vi "Configure Connection Dialog.vi"(8 "error in (no error)":errorcluster, 10 "Current Connection":T8, 11 "Channel Editor State":T1={"Modules and Connections"=[{" Module Path"="", "Short Module Path"="", "Product Name"="", "Possible Connections"=[], "Missing"=FALSE}, {" Module Path"="", "Short Module Path"="", "Product Name"="", "Possible Connections"=[], "Missing"=FALSE}], "Alias Mappings UI"=[], "Mappings by Module UI"=[]}) -> (0 "error out":errorcluster, 1 "Connection (R,S,D)":T7, 2 "Canceled?":bool)   [LabVIEW 2020, in "Routing and Faulting System Explorer.lvlib"]
uses:
  Routing and Faulting System Explorer.lvlib
  Connection Row.ctl
  Shared/Connection.ctl
  Channel Editor State.ctl
  Possible Connections.ctl
  Shared/Routing and Faulting Hardware API/Types/Possible Connections for Endpoint.ctl
  Shared/Alias Mapping.ctl
  Shared/Alias Endpoint.ctl
  Alias Map by Module.ctl
  <vilib>/event_ctls.llb/lveventtype.ctl
  Shared/Constants.vi
  Shared/Routing and Faulting Shared.lvlib
  Shared/Routing and Faulting Hardware API/Routing and Faulting Hardware API.lvlib
panel:
  out "Product Name List":string[](array[string])
  out "Module Index":i32
  out "Initial Module":string
  out "Initial Destination":string
  out "Initial Source":string
  in  "Module":string(combo)
  in  "Cancel Button":bool
  in  "OK Button":bool
  in  "Destination":string(combo)
  in  "Source":string(combo)
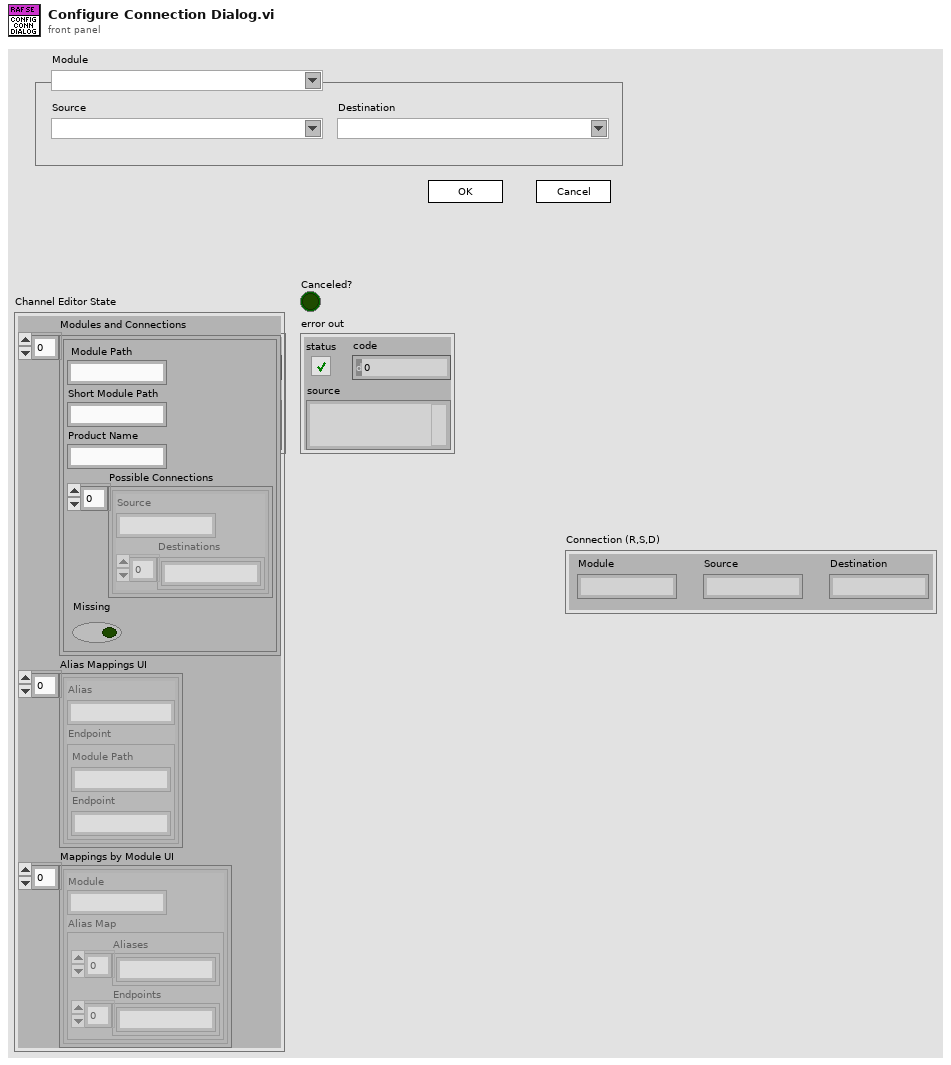
[diagram p1: front panel]
types:
  T1 = typedef "Routing and Faulting System Explorer.lvlib/Channel Editor State.ctl" = cluster{"Modules and Connections":T2[], "Alias Mappings UI":T4[], "Mappings by Module UI":T6[]}
  T2 = typedef "Routing and Faulting System Explorer.lvlib/Possible Connections.ctl" = cluster{" Module Path":string, "Short Module Path":string, "Product Name":string, "Possible Connections":T3[], "Missing":bool}
  T3 = typedef "Routing and Faulting Hardware API.lvlib/Possible Connections for Endpoint.ctl" = cluster{"Source":string, "Destinations":string[]}
  T4 = typedef "Routing and Faulting Shared.lvlib/Alias Mapping.ctl" = cluster{"Alias":string, "Endpoint":T5}
  T5 = typedef "Routing and Faulting Shared.lvlib/Alias Endpoint.ctl" = cluster{"Module Path":string, "Endpoint":string}
  T6 = typedef "Routing and Faulting System Explorer.lvlib/Alias Map by Module.ctl" = cluster{"Module":string, "Alias Map":cluster{"Aliases":string[], "Endpoints":string[]}}
  T7 = typedef "Routing and Faulting Shared.lvlib/Connection.ctl" = cluster{"Module":string, "Source":string, "Destination":string}
  T8 = typedef "Routing and Faulting System Explorer.lvlib/Connection Row.ctl" = cluster{"Source":string, "Destination":string, "Edit":bool, "Remove":bool}
  T9 = typedef "lveventtype.ctl" = enum32{"Null", "Timeout", "Annotation Menu Selection", "Annotation Menu Selection?", "App Instance Close", "App Instance Close?", "Autoscale Range Change", "Bookmark Info Change", "Cell Edit", "Cell Edit?", "Cursor Grab", "Cursor Grab?", "Cursor Menu Selection", "Cursor Menu Selection?", "Cursor Move", "Cursor Release", "Data Change", "Direction Change", "Display State Change", "Drag Ended", "Drag Enter", "Drag Leave", "Drag Over", "Drag Source Update", "Drag Starting", "Drag Starting?", "Drop", "Exec State Change", "Key Down", "Key Down?", "Key Repeat", "Key Repeat?", "Key Up", "Listbox Double Click", "Menu Activation?", "Menu Selection (App)", "Menu Selection? (App)", "Menu Selection (User)", "Mouse Down", "Mouse Down?", "Mouse Enter", "Mouse Leave", "Mouse Move", "Mouse Up", "Mouse Wheel", "NI Security User Change (App)", "Pane Size", "Panel Close", "Panel Close?", "Panel Resize", "Plot Attribute Change", "Scale Range Change", "Shortcut Menu Activation?", "Shortcut Menu Selection (App)", "Shortcut Menu Selection? (App)", "Shortcut Menu Selection (User)", "Tree Double Click", "Tree Drag", "Tree Drag?", "Tree Drop", "Tree Drop?", "Tree Item Close", "Tree Item Close?", "Tree Item Open", "Tree Item Open?", "User Event", "Value Change"}
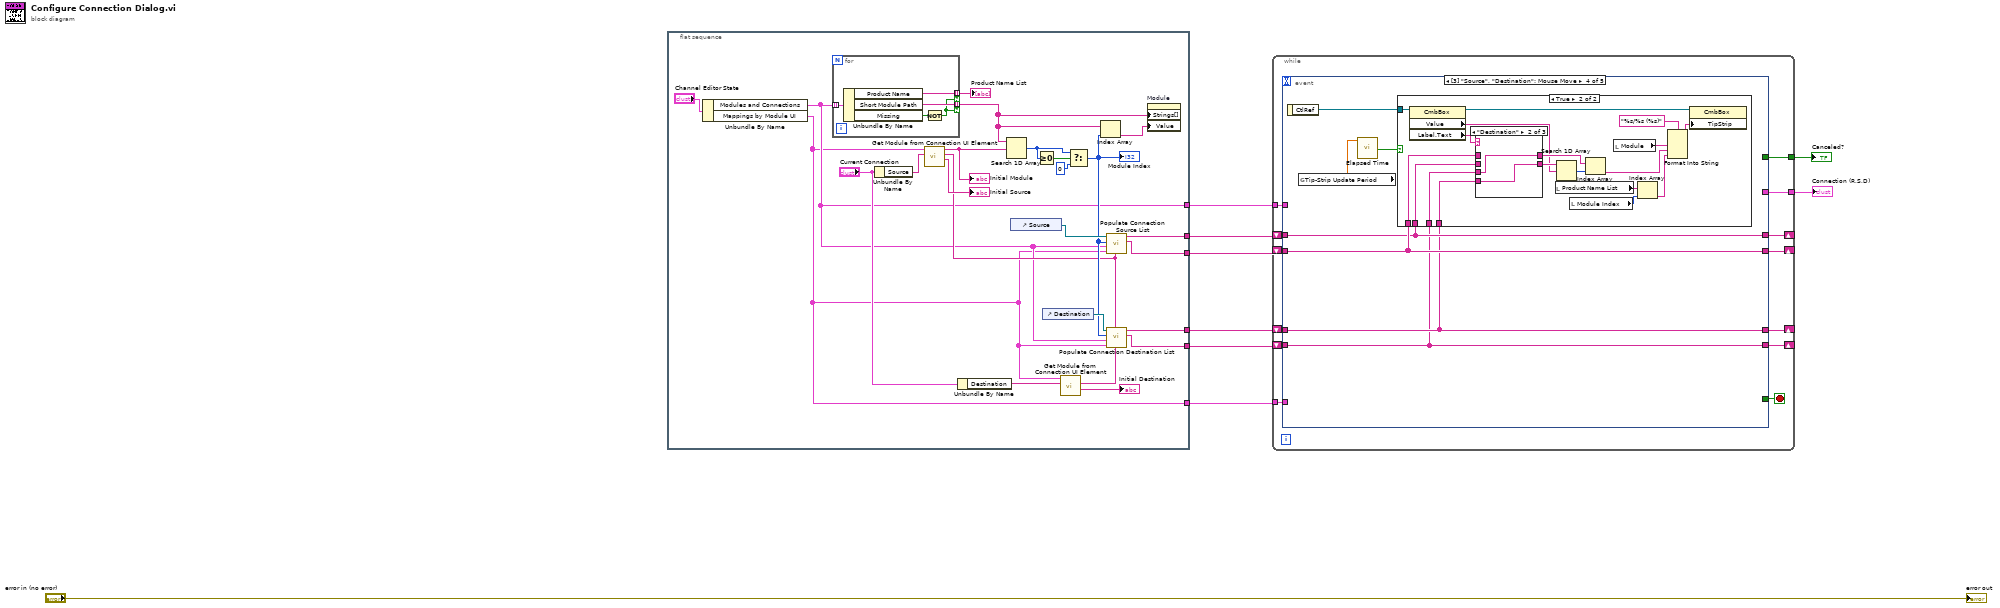
[diagram p0: block diagram]
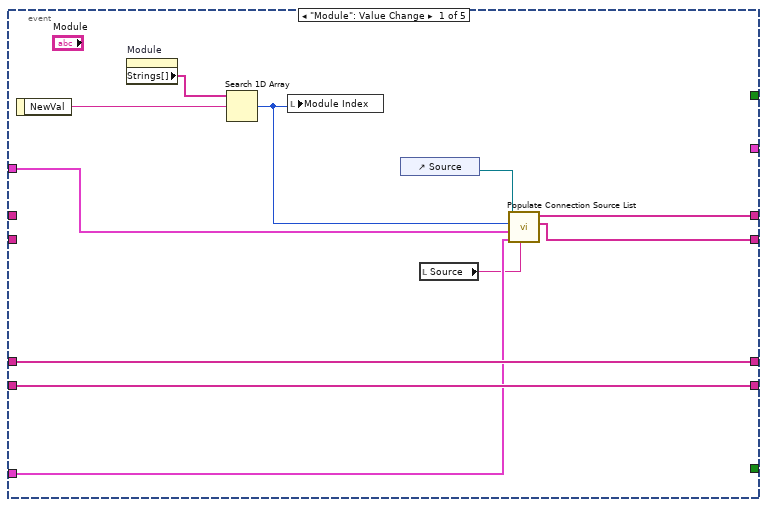
[diagram p2: hidden frame]
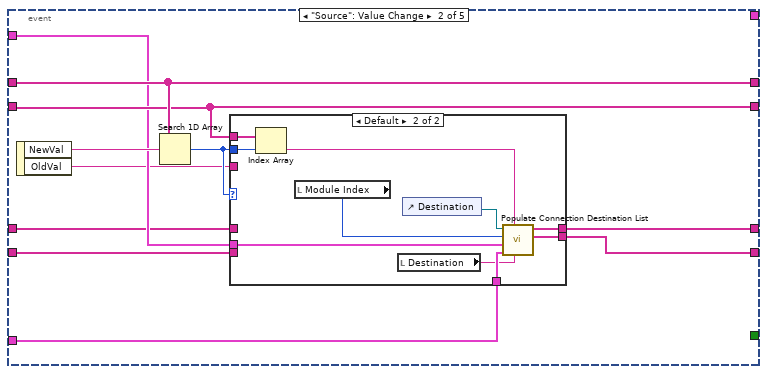
[diagram p3: hidden frame]
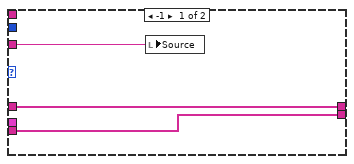
[diagram p4: hidden frame]
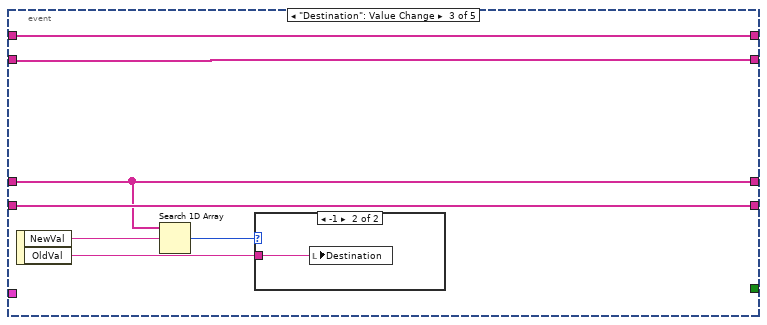
[diagram p5: hidden frame]
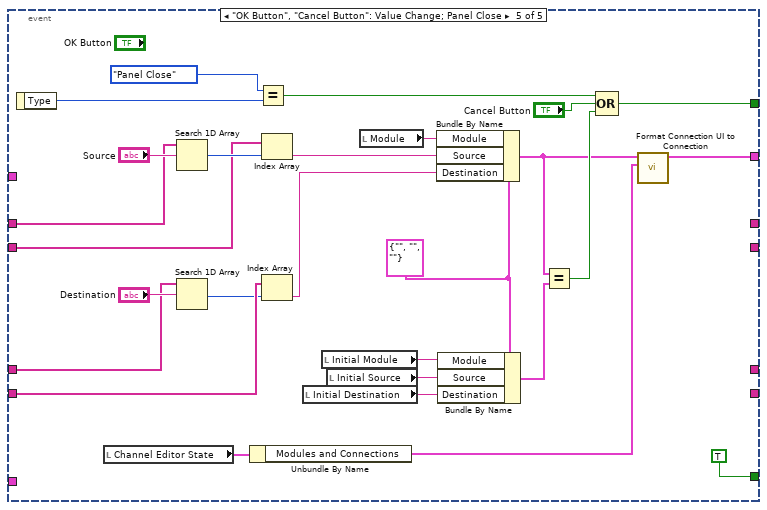
[diagram p10: hidden frame]
diagram:
  n1 = flat-sequence {
    tunnel: [w29] -> w7
    tunnel: [w11] -> w2
    tunnel: [w26] -> w6
    tunnel: [w25] -> w5
    tunnel: [w12] -> w4
    tunnel: [w28] -> w3
    frame #0 {
      n2 = Unbundle By Name("Channel Editor State") -> ("Modules and Connections"=w12:T2[], "Mappings by Module UI"=w11:T6[])
      n3 = for {
        tunnel: w12 -> [w38] mode=indexing
        tunnel: [w37] -> w33 mode=indexing if=w34
        tunnel: [w36] -> w10 mode=indexing if=w34
        n4 = Unbundle By Name(w38) -> ("Product Name"=w36:string, "Short Module Path"=w37:string, "Missing"=w35:bool)
        n5 = Not(x=w35) -> (.not. x?=w34:bool)
      }
      "Product Name List" <- w10
      n6 = Unbundle By Name("Current Connection") -> ("Source"=w19:string)
      n7 = call "Get Module from Connection UI Element.vi"("Alias or Full Endpoint"=w19, "Alias Mappings by Module"=w11) -> ("Long Endpoint"=→"Initial Source":string, "Short Endpoint"=w17:string, "Module"=w31:string)  [unwired: 7 in]
      "Initial Module" <- w31
      n8 = Unbundle By Name("Current Connection") -> ("Destination"=w16:string)
      n9 = Search 1D Array(1D array=w33, element=w31) -> (index of element=w23:i32)  [unwired: 1 in]
      n10 = control-ref of="Source"() -> (w30:refnum<vi>)
      n11 = Greater Or Equal To 0?(x=w23) -> (x >= 0?=w24:bool)
      n12 = control-ref of="Destination"() -> (w27:refnum<vi>)
      n13 = call "Get Module from Connection UI Element.vi"("Alias or Full Endpoint"=w16, "Alias Mappings by Module"=w11) -> ("Long Endpoint"=→"Initial Destination":string, "Short Endpoint"=w14:string)  [unwired: 7 in, 1 out]
      n14 = Select(t=w23, s=w24, f=0) -> (s? t:f=w20:i32)
      "Module Index" <- w20
      n15 = Index Array(array=w33, index=w20) -> (element=w32:string)
      n16 = call "Populate Connection Source List.vi"("initial Source"=w17, "Alias Mappings by Module"=w11, "Possible Connections"=w12, "Module Index"=w20, "Source Reference"=w30) -> ("Endpoint List"=w28:string[], "Alias List"=w29:string[])  [unwired: 5 in]
      n17 = call "Populate Connection Destination List.vi"("initial Destination"=w14, "Source"=w17, "Alias Mappings by Module"=w11, "Possible Connections"=w12, "Module Index"=w20, "Destination Reference"=w27) -> ("Endpoint List"=w25:string[], "Alias List"=w26:string[])  [unwired: 4 in]
      n18 = property on="Module" class="CmbBox"("Strings[]"=w33, "Value"=w32) -> ()  [unwired: 2 in, 2 out]
    }
  }
  n19 = while {
    tunnel: [w50] -> w9
    tunnel: w4 -> [w49]
    shift-right: [w45] -> _
    shift-left: w7 -> [w48]
    shift-right: [w44] -> _
    shift-left: w3 -> [w47]
    tunnel: w2 -> [w46]
    shift-right: [w43] -> _
    shift-left: w6 -> [w41]
    shift-right: [w42] -> _
    shift-left: w5 -> [w40]
    tunnel: [w39] -> w1
    stop <- w51 stop-if-true
    n20 = event shown="[3] \"Source\", \"Destination\": Mouse Move" {
      selector: _ -> [_ _ _ _ _]
      dyn-events: _ -> [_ _ _ _ _]
      timeout: _ -> [_ _ _ _ _]
      tunnel: [_ _ _ _ TRUE] -> w51
      tunnel: [_ _ _ _ w146] -> w50
      tunnel: w49 -> [w55 w68 _ _ _]
      tunnel: w48 -> [_ w72 w92 w100 w142]
      tunnel: w47 -> [_ w69 w91 w101 w141]
      tunnel: w46 -> [w56 w67 _ _ _]
      tunnel: [w61 w72 w92 w100 _] -> w45
      tunnel: [w60 w69 w91 w101 _] -> w44
      tunnel: [w59 w71 w89 w99 _] -> w43
      tunnel: [w58 w70 w90 w98 _] -> w42
      tunnel: w41 -> [w59 w65 w89 w99 w138]
      tunnel: w40 -> [w58 w64 w90 w98 w137]
      tunnel: [_ _ _ _ w124] -> w39
      event "Module": Value Change {
        n21 = event-data() -> ("NewVal"=w62:string)  [unwired: 1 in]
        n22 = property on="Module" class="CmbBox"() -> ("Strings[]"=w54:string[])  [unwired: 2 in, 2 out]
        n23 = Search 1D Array(1D array=w54, element=w62) -> (index of element=w53:i32)  [unwired: 1 in]
        n24 = local write "Module Index"(w53) -> ()
        n25 = control-ref of="Source"() -> (w57:refnum<vi>)
        n26 = local read "Source"() -> (w52:string)
        n27 = call "Populate Connection Source List.vi"("initial Source"=w52, "Alias Mappings by Module"=w56, "Possible Connections"=w55, "Module Index"=w53, "Source Reference"=w57) -> ("Endpoint List"=w60:string[], "Alias List"=w61:string[])  [unwired: 5 in]
      }
      event "Source": Value Change {
        n28 = event-data() -> ("NewVal"=w73:string, "OldVal"=w63:string)  [unwired: 1 in]
        n29 = Search 1D Array(1D array=w72, element=w73) -> (index of element=w66:i32)  [unwired: 1 in]
        n30 = case shown="Default" w66 {
          tunnel: w66 -> [_ w86]
          tunnel: [w76 w85] -> w71
          tunnel: [w75 w84] -> w70
          tunnel: w69 -> [_ w83]
          tunnel: w68 -> [_ w81]
          tunnel: w67 -> [_ w79]
          tunnel: w65 -> [w76 _]
          tunnel: w64 -> [w75 _]
          tunnel: w63 -> [w74 _]
          frame -1 {
            n31 = local write "Source"(w74) -> ()
          }
          frame Default {
            n32 = Index Array(array=w83, index=w86) -> (element=w78:string)
            n33 = local read "Module Index"() -> (w82:i32)
            n34 = local read "Destination"() -> (w77:string)
            n35 = control-ref of="Destination"() -> (w80:refnum<vi>)
            n36 = call "Populate Connection Destination List.vi"("initial Destination"=w77, "Source"=w78, "Alias Mappings by Module"=w79, "Possible Connections"=w81, "Module Index"=w82, "Destination Reference"=w80) -> ("Endpoint List"=w84:string[], "Alias List"=w85:string[])  [unwired: 4 in]
          }
        }
      }
      event "Destination": Value Change {
        n37 = event-data() -> ("NewVal"=w93:string, "OldVal"=w87:string)  [unwired: 1 in]
        n38 = Search 1D Array(1D array=w89, element=w93) -> (index of element=w88:i32)  [unwired: 1 in]
        n39 = case shown="-1" w88 {
          tunnel: w87 -> [_ w94]
          frame Default {
          }
          frame -1 {
            n40 = local write "Destination"(w94) -> ()
          }
        }
      }
      event "Source", "Destination": Mouse Move {
        n41 = event-data() -> ("CtlRef"=w97:refnum<vi>)  [unwired: 1 in]
        n42 = global read "Constants.vi" "Tip-Strip Update Period"() -> (w96:dbl)
        n43 = call "Elapsed Time"("Time Target (s)"=w96) -> ("Time has Elapsed"=w95:bool)  [unwired: 11 in, 7 out]
        n44 = case shown="True" w95 {
          tunnel: w101 -> [_ w111]
          tunnel: w100 -> [_ w110]
          tunnel: w99 -> [_ w109]
          tunnel: w98 -> [_ w108]
          tunnel: w97 -> [_ w104]
          frame False {
            # "Only process mouse moves every 10ms"
          }
          frame True {
            n45 = property class="CmbBox"(reference=w104) -> (reference out=w103:refnum<vi>, "Value"=w102:string, "Label.Text"=w105:string)  [unwired: 1 in, 1 out]
            n46 = case shown="\"Destination\"" w105 {
              tunnel: w111 -> [w120 _ _]
              tunnel: w110 -> [w121 _ _]
              tunnel: w109 -> [_ w123 _]
              tunnel: w108 -> [_ w122 _]
              tunnel: [w121 w123 _] -> w107
              tunnel: [w120 w122 _] -> w106
              frame "Source" {
              }
              frame "Destination" {
              }
              frame Default {
              }
            }
            n47 = local read "Product Name List"() -> (w115:string[])
            n48 = Search 1D Array(1D array=w107, element=w102) -> (index of element=w119:i32)  [unwired: 1 in]
            n49 = local read "Module Index"() -> (w114:i32)
            n50 = Index Array(array=w106, index=w119) -> (element=w116:string)
            n51 = local read "Module"() -> (w117:string)
            n52 = Index Array(array=w115, index=w114) -> (element=w113:string)
            n53 = Format Into String(format string="%s/%s (%s)", w117, w116, w113) -> (resulting string=w112:string)  [unwired: 2 in, 1 out]
            n54 = property class="CmbBox"(reference=w103, "TipStrip"=w112) -> ()  [unwired: 1 in, 2 out]
          }
        }
      }
      event "OK Button", "Cancel Button": Value Change; Panel Close {
        w134 = T7 {"Module"="", "Source"="", "Destination"=""} ("Connection (R,S,D)")
        n55 = event-data() -> ("Type"=w148:T9)  [unwired: 1 in]
        n56 = local read "Channel Editor State"() -> (w127:T1)
        n57 = Search 1D Array(1D array=w142, element="Source") -> (index of element=w144:i32)  [unwired: 1 in]
        n58 = Search 1D Array(1D array=w138, element="Destination") -> (index of element=w136:i32)  [unwired: 1 in]
        n59 = Unbundle By Name(w127) -> ("Modules and Connections"=w125:T2[])
        n60 = Equal?(x=lveventtype."Panel Close" ("Type"), y=w148) -> (x = y?=w129:bool)
        n61 = Index Array(array=w141, index=w144) -> (element=w140:string)
        n62 = Index Array(array=w137, index=w136) -> (element=w135:string)
        n63 = local read "Initial Destination"() -> (w130:string)
        n64 = local read "Initial Module"() -> (w132:string)
        n65 = local read "Initial Source"() -> (w131:string)
        n66 = local read "Module"() -> (w145:string)
        n67 = Bundle By Name(cluster=w134, "Module"=w145, "Source"=w140, "Destination"=w135) -> (w126:T7)
        n68 = Bundle By Name(cluster=w134, "Module"=w132, "Source"=w131, "Destination"=w130) -> (w133:T7)
        n69 = Equal?(x=w126, y=w133) -> (x = y?=w128:bool)
        n70 = Compound Arithmetic op=OR(w129, "Cancel Button", w128) -> (w146:bool)
        n71 = call "Format Connection UI to Connection.vi"("Modules and Connections"=w125, "Connection UI"=w126) -> ("Connection"=w124:T7)  [unwired: 9 in]
      }
    }
  }
  "Canceled?" <- w9
  "Connection (R,S,D)" <- w1
  "error out" <- "error in (no error)"
